vi "Get Components Target Directory.vi"(8 "error in (no error)":errorcluster, 11 "Item Ref in":T1 format="%.0x") -> (0 "error out":errorcluster, 2 "components target directory":path, 3 "Item Ref out":T1 format="%.0x")   [LabVIEW 2017, in "DSF Shared.lvlib"]
uses:
  DSF Shared.lvlib
  <vilib>/NI Veristand/Custom Device API/Custom Device Item Ref.ctl
  <vilib>/NI Veristand/Custom Device API/Get Item Property (Path).vi
  <vilib>/NI Veristand/Custom Device API/Custom Device API.lvlib
  System Explorer/DSF System Explorer.lvlib
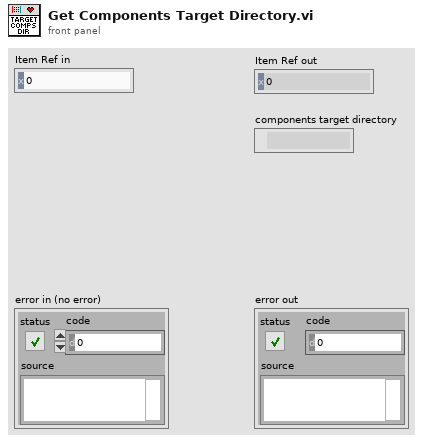
[diagram p1: front panel]
types:
  T1 = typedef "Custom Device API.lvlib/Custom Device Item Ref.ctl" = u64
  T2 = typedef "Custom Device API.lvlib/Custom Device Target Type.ctl" = enum16{"PharLap", "VxWorks", "Windows", "Linux_32_ARM", "Linux_x64"}
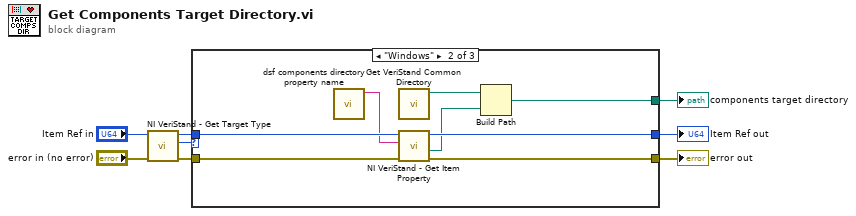
[diagram p0: block diagram]
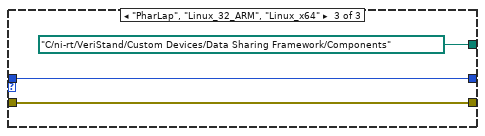
[diagram p3: hidden frame]
diagram:
  n1 = call <vilib>:"NI VeriStand - Get Target Type.vi"("error in (no error)"="error in (no error)", "Item Ref in"="Item Ref in") -> ("error out"=w4:errorcluster, "Target Type"=w6:T2, "Item Ref out"=w5:T1)  [unwired: 7 in]
  n2 = case shown="\"Windows\"" w6 {
    tunnel: w5 -> [w10 w18 w20]
    tunnel: w4 -> [w9 w17 w21]
    tunnel: [_ w11 path "C:/ni-rt/VeriStand/Custom Devices/Data Sharing Framework/Components" ("RT Destination")] -> w3
    tunnel: [w9 w15 w21] -> w2
    tunnel: [w10 w16 w20] -> w1
    frame Default {
    }
    frame "Windows" {
      n3 = call "dsf components directory property name.vi"() -> ("components directory property name"=w14:string)  [unwired: 11 in]
      n4 = call "Get VeriStand Common Directory.vi"() -> ("common directory"=w13:path)  [unwired: 11 in]
      n5 = call-poly <vilib>:"NI VeriStand - Get Item Property.vi"("error in (no error)"=w17, "Property Name"=w14, "Item Ref in"=w18) -> ("error out"=w15:errorcluster, "Value"=w12:path, "Item Ref out"=w16:T1)  [unwired: 5 in, 1 out]
      n6 = Build Path(base path=w13, name or relative path=w12) -> (appended path=w11:path)
    }
    frame "PharLap", "Linux_32_ARM", "Linux_x64" {
    }
  }
  "Item Ref out" <- w1
  "error out" <- w2
  "components target directory" <- w3
